vi "SFC_After Burning.vi"(0 "Traceability 引用句柄":refnum<k24>, 1 "Positon":string, 2 "UserNo":string, 5 "IntSN":string, 7 "Process":string, 9 "testResult":string, 11 "error in (no error)":errorcluster caption="错误输入（无错误）", 12 "BurnTime":dbl) -> (4 "Traceability 引用句柄输出":refnum<k24>, 6 "SFC_AfterBurning":string, 15 "error out":errorcluster caption="错误输出")   [LabVIEW 2014, in "Traceability.lvlib"]
uses:
  D:/webservice/Traceability.dll
  Traceability.dll
  Traceability.lvlib
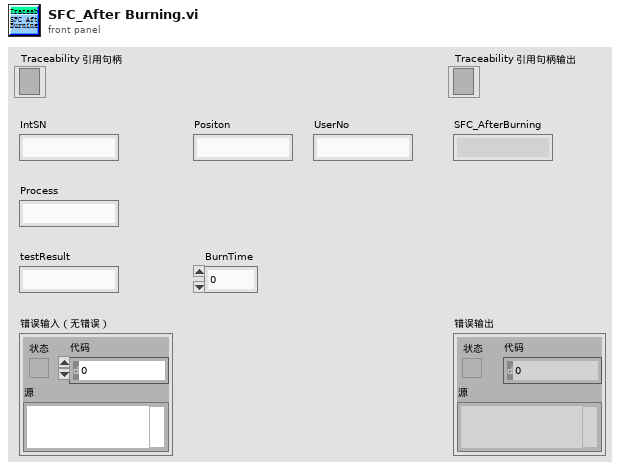
[diagram p1: front panel]
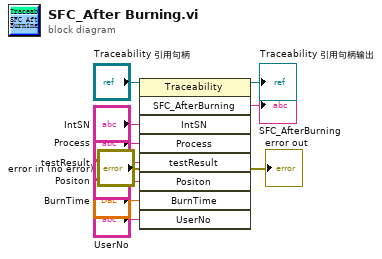
[diagram p0: block diagram]
diagram:
  n1 = invoke class="Traceability" method="SFC_AfterBurning"(reference="Traceability 引用句柄", error in="error in (no error)", "IntSN"="IntSN", "Process"="Process", "testResult"="testResult", "Positon"="Positon", "BurnTime"="BurnTime", "UserNo"="UserNo") -> (reference out=→"Traceability 引用句柄输出":refnum<k24>, error out=→"error out":errorcluster, "SFC_AfterBurning"=→"SFC_AfterBurning":string)  [unwired: 1 in, 6 out]
